vi "Start Continuous Test Cycles (No Data) [STL].vi"(7 "Micropulse # In":i32, 8 "error in (no error)":errorcluster, 11 "Test Number":u32=1 caption="Test Number (1 to 1279)" min=1 max=1279) -> (0 "error out":errorcluster, 5 "Micropulse # Out":i32)   [LabVIEW 2026, in "MicroPulse_Driver.lvlib"]
doc: "To perform specified test without data output.\n\nAny previously selected inspection mode is terminated, and any driven axis is stopped. The requested test is displayed on the A-scan monitor (if available)\n\nParameters:\n<Tn>: Number of the test to be performed.\nAn Integer value from 1 to the maximum number of tests (default maximum is 1279)"
uses:
  MicroPulse_Driver.lvlib
  Private/MP-Registry Action-Enum.ctl
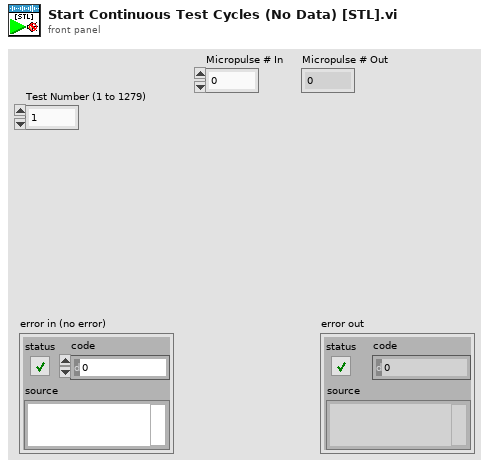
[diagram p1: front panel]
types:
  T1 = typedef "MicroPulse_Driver.lvlib/TCP config.ctl" = cluster{"Connection ID":refnum<k5>, "IP address":string, "host port":u16, "OC timeout":i32, "Read timeout":i32, "Write timeout":i32}
  T2 = typedef "MicroPulse_Driver.lvlib/MP-Registry Action-Enum.ctl" = enum16{"Read", "Add Test", "Add Command", "Add Gate Command", "Add Encoder Command", "Clear Command  List", "Set Registry", "Set System Details", "Set DOF", "Set Velocity", "Disable Asynch Reads", "Enable Asynch Reads", "Add Connection", "Disconnect", "Shutdown"}
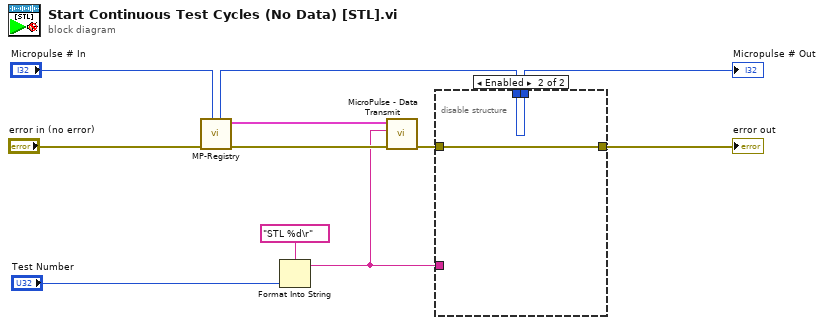
[diagram p0: block diagram]
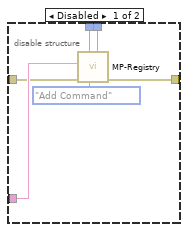
[diagram p2: hidden frame]
diagram:
  n1 = call "MP-Registry.vi"("Micropulse # In"="Micropulse # In", "error in (no error)"="error in (no error)") -> ("error out"=w9:errorcluster, "TCP config"=w8:T1, "Micropulse # Out"=w3:i32)  [unwired: 6 in, 1 out]
  n2 = Format Into String(format string="STL %d\r", "Test Number") -> (resulting string=w6:string)  [unwired: 2 in, 1 out]
  n3 = call "MicroPulse - Data Transmit.vi"("error in (no error)"=w9, "data"=w6, "TCP config"=w8) -> ("error out"=w5:errorcluster)  [unwired: 6 in, 2 out]
  n4 = disable-structure shown="Enabled" {
    disable-tunnel: w6 -> [w17 _]
    disable-tunnel: w5 -> [w15 w18]
    disable-tunnel: [w14 w18] -> w4
    disable-tunnel: w3 -> [w13 w19]
    disable-tunnel: [w12 w19] -> w2
    frame Disabled {
      n5 = call "MP-Registry.vi"("Action"=MP-Registry_Action-Enum."Add Command", "Micropulse # In"=w13, "error in (no error)"=w15, "Data in"=w17) -> ("error out"=w14:errorcluster, "Micropulse # Out"=w12:i32)  [unwired: 4 in, 2 out]
    }
    frame Enabled {
    }
  }
  "error out" <- w4
  "Micropulse # Out" <- w2
